vi "iTricubeWeights.vi"(1 "Array":dbl[](array[numeric])) -> (0 "Weights":dbl[](array[numeric]))   [LabVIEW 2020]
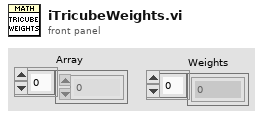
[diagram p1: front panel]
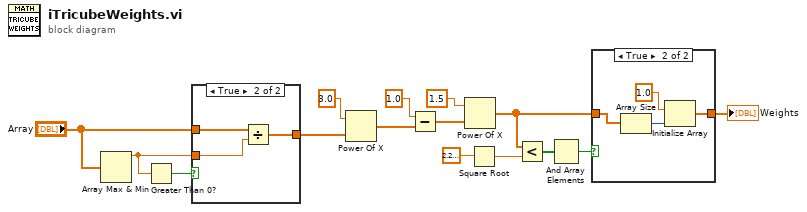
[diagram p0: block diagram]
diagram:
  n1 = Array Max & Min(array="Array") -> (max value=w13:dbl)  [unwired: 3 out]
  n2 = Greater Than 0?(x=w13) -> (x > 0?=w15:bool)
  n3 = case shown="True" w15 {
    tunnel: "Array" -> [w16 w19]
    tunnel: w13 -> [_ w18]
    tunnel: [w16 w17] -> w12
    frame False {
    }
    frame True {
      n4 = Divide(x=w19, y=w18) -> (x/y=w17:dbl[])
    }
  }
  n5 = Power Of X(1:w12, 2:3.0) -> (0:w10:dbl[])
  n6 = Subtract(x=1.0, y=w10) -> (x-y=w8:dbl[])
  n7 = Power Of X(1:w8, 2:1.5) -> (0:w2:dbl[])
  n8 = Square Root(x=2.220446049250313e-16) -> (sqrt(x)=w5:dbl)
  n9 = Less?(x=w2, y=w5) -> (x < y?=w4:bool[])
  n10 = And Array Elements(Boolean array=w4) -> (logical AND=w3:bool)
  n11 = case shown="True" w3 {
    tunnel: w2 -> [w20 w23]
    tunnel: [w20 w24] -> w1
    frame False {
    }
    frame True {
      n12 = Array Size(array=w23) -> (size(s)=w22:i32)
      n13 = Initialize Array(1.0, w22) -> (w24:dbl[])
    }
  }
  "Weights" <- w1
